vi "SS2 Live_Refresh Single Parameter.vi"(7 "Verbose (T)":bool=TRUE, 8 "Error In":errorcluster, 9 "Data":variant, 10 "Control Label":string, 11 "VI Ref in":refnum<vi>) -> (0 "Error Out":errorcluster)   [LabVIEW 2019]
panel:
  out "Owning Tab Name":string
  out "Ctl found?":bool
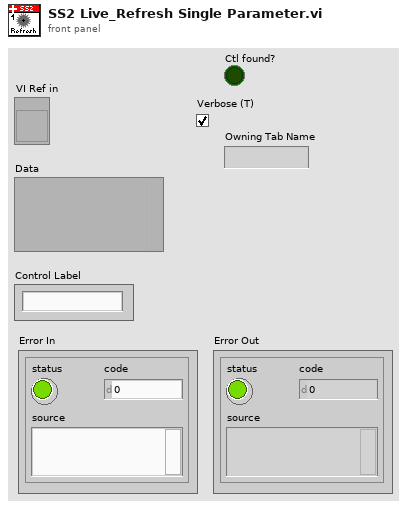
[diagram p1: front panel]
types:
  T1 = enum16{"Controls & Indicators", "Controls", "Indicators"}
  T2 = typedef "SS2 Live_Settings List.ctl" = enum16{"FPGA:Bitfile Path", "FPGA:Bitfile Version", "Acquisition Parameters:SS2 DAQ Parameters", "Acquisition Parameters:Gate Configuration Array", "Acquisition Parameters:Buffer Size (# Gates)", "File Information:File Information", "File Information:# Datasets in Series", "Image Parameters:Image ROI Information", "Image Parameters:Image Binning Options", "UI Parameters:Histogram Bins Number"}
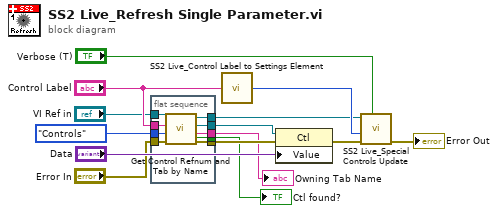
[diagram p0: block diagram]
diagram:
  n1 = flat-sequence {
    tunnel: "Control Label" -> [w23]
    tunnel: [w22] -> w12
    tunnel: [w21] -> w9
    tunnel: [w20] -> w8
    tunnel: T1."Controls" ("Selection") -> [w19]
    tunnel: "VI Ref in" -> [w18]
    tunnel: "Error In" -> [w17]
    tunnel: [w16] -> w2
    tunnel: [w15] -> w1
    frame #0 {
      n2 = call "Get Control Refnum and Tab by Name.vi"("error in"=w17, "Selection"=w19, "Control Label"=w23, "VI  Ref"=w18) -> ("error out"=w21:errorcluster, "Owning Tab Name"=w15:string, "Ctl Refnum"=w20:refnum<vi>, "VI  Ref (out)"=w22:refnum<vi>, "Ctl found?"=w16:bool)  [unwired: 3 in]
    }
  }
  n3 = call "SS2 Live_Control Label to Settings Element.vi"("Control Label"="Control Label") -> ("Settings List Element"=w14:T2)  [unwired: 8 in]
  n4 = property class="Ctl"(reference=w8, error in=w9, "Value"="Data") -> (error out=w11:errorcluster)  [unwired: 1 out]
  n5 = call "SS2 Live_Special Controls Update.vi"("Verbose (T)"="Verbose (T)", "error in (no error)"=w11, "Settings List Element"=w14, "VI Refnum"=w12) -> ("Error Out"=→"Error Out":errorcluster)  [unwired: 7 in]
  "Ctl found?" <- w2
  "Owning Tab Name" <- w1
